vi "test6-AsyncMessageWithReplyWithError.vi"(8 "error in (no error)":errorcluster, 11 "TestCase in":refnum<class "testcase-CSMMessage.lvclass">) -> (0 "error out":errorcluster, 3 "TestCase out":refnum<class "testcase-CSMMessage.lvclass">)   [LabVIEW 2017, in "testcase-CSMMessage.lvclass"]
uses:
  testcase-CSMMessage.lvclass
  948582eb-d69d-4bf1-bb36-25d021f5d5c5.vi
  src/user.lib/_NEVSTOP/Communicable State Machine(CSM)/AdvanceAPI/CSM - Make String Arguments Safe.vi
  src/user.lib/_NEVSTOP/Communicable State Machine(CSM)/AdvanceAPI/CSM - Keywords.vi
  <vilib>/addons/_JKI Toolkits/VI Tester/TestCase.llb/TestCase.lvclass
  src/user.lib/_NEVSTOP/Communicable State Machine(CSM)/Communicable State Machine.lvlib
  C:/Program Files (x86)/National Instruments/LabVIEW 2017/vi.lib/addons/_JKI Toolkits/VI Tester/TestCase.llb/TestCase.lvclass
panel:
  out "Loop Count":i32
  out "concatenated string":string
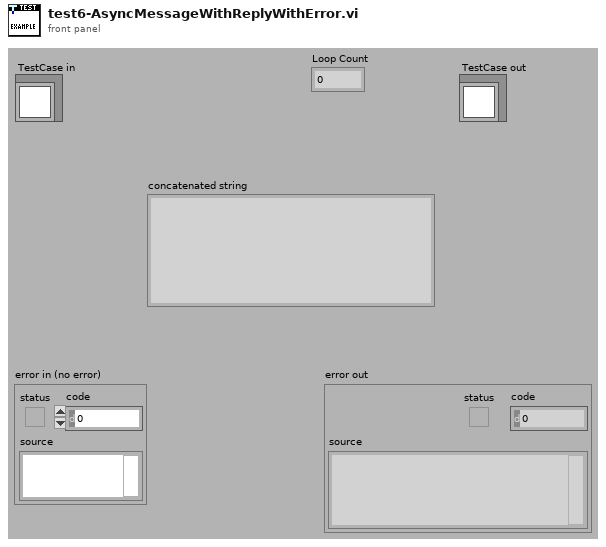
[diagram p1: front panel]
types:
  T1 = cluster{"Arguments":string, "Response":string, "error":errorcluster}
  T2 = cluster{"status":bool, "code":bool, "source":bool}
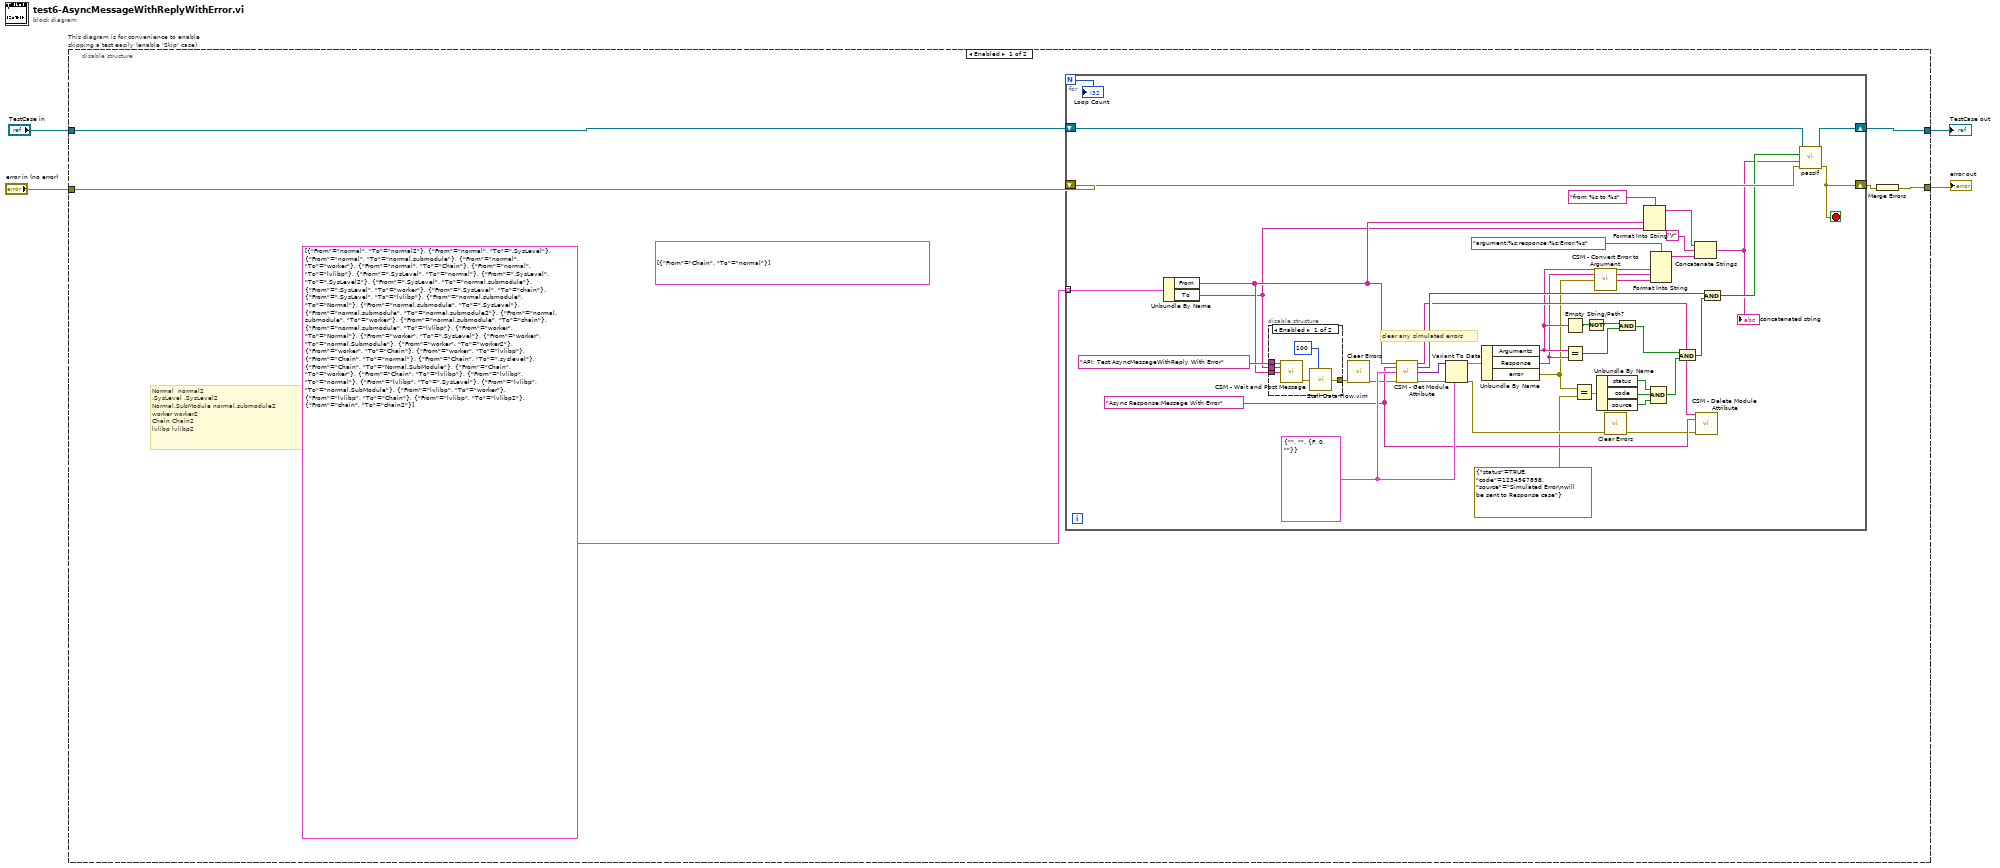
[diagram p0: block diagram]
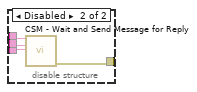
[diagram p2: hidden frame]
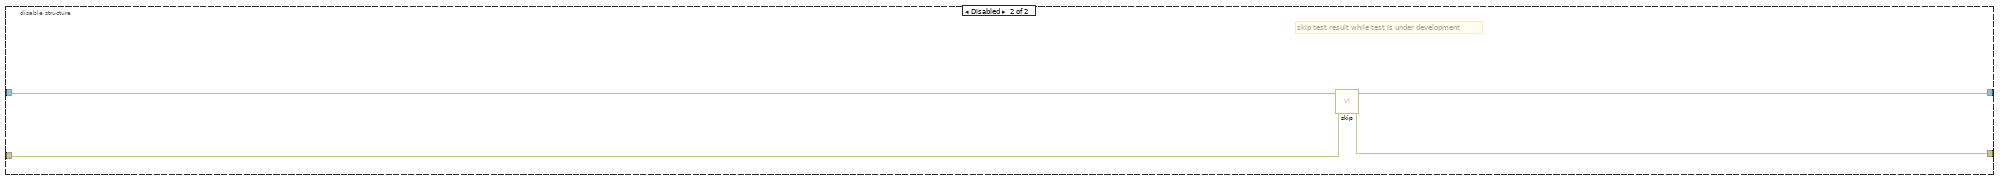
[diagram p3: hidden frame]
diagram:
  n1 = disable-structure "This diagram is for convenience to enable skipping a test easily (enable 'Skip' case)" shown="Enabled" {
    disable-tunnel: "TestCase in" -> [w10 w66]
    disable-tunnel: [w9 w64] -> w1
    disable-tunnel: [w6 w65] -> w3
    disable-tunnel: "error in (no error)" -> [w7 w63]
    frame Enabled {
      (unwired) cluster{"From":string, "To":string}[] [{"From"="Chain", "To"="normal"}]
      # "Normal  normal2\n.SysLevel .SysLevel2\nNormal.SubModule normal.submodule2\nworker worker2\nChain Chain2\nlvlibp lvlibp2"
      n2 = for {
        N -> [w11]
        tunnel: cluster{"From":string, "To":string}[] [{"From"="normal", "To"="normal2"}, {"From"="normal", "To"=".SysLevel"}, {"From"="normal", "To"="normal.submodule"}, {"From"="normal", "To"="worker"}, {"From"="normal", "To"="Chain"}, {"From"="normal", "To"="lvlibp"}, {"From"=".SysLevel", "To"="normal"}, {"From"=".SysLevel", "To"=".SysLevel2"}, {"From"=".SysLevel", "To"="normal.submodule"}, {"From"=".SysLevel", "To"="worker"}, {"From"=".SysLevel", "To"="chain"}, {"From"=".SysLevel", "To"="lvlibp"}, {"From"="normal.submodule", "To"="Normal"}, {"From"="normal.submodule", "To"=".SysLevel"}, {"From"="normal.submodule", "To"="normal.submodule2"}, {"From"="normal.submodule", "To"="worker"}, {"From"="normal.submodule", "To"="chain"}, {"From"="normal.submodule", "To"="lvlibp"}, {"From"="worker", "To"="Normal"}, {"From"="worker", "To"=".SysLevel"}, {"From"="worker", "To"="normal.Submodule"}, {"From"="worker", "To"="worker2"}, {"From"="worker", "To"="Chain"}, {"From"="worker", "To"="lvlibp"}, {"From"="Chain", "To"="normal"}, {"From"="Chain", "To"=".syslevel"}, {"From"="Chain", "To"="Normal.SubModule"}, {"From"="Chain", "To"="worker"}, {"From"="Chain", "To"="lvlibp"}, {"From"="lvlibp", "To"="normal"}, {"From"="lvlibp", "To"=".SysLevel"}, {"From"="lvlibp", "To"="normal.SubModule"}, {"From"="lvlibp", "To"="worker"}, {"From"="lvlibp", "To"="Chain"}, {"From"="lvlibp", "To"="lvlibp2"}, {"From"="chain", "To"="chain2"}] -> [w41] mode=indexing
        shift-right: [w51] -> w9
        shift-left: w10 -> [w52]
        shift-right: [w23] -> w8
        shift-left: w7 -> [w50]
        stop <- w23 stop-if-true
        w47 = T1 {"Arguments"="", "Response"="", "error"={"status"=FALSE, "code"=0, "source"=""}}
        w38 = "Async Response:Message With Error" ("State")
        # "clear any simulated errors"
        n3 = Unbundle By Name(w41) -> ("From"=w15:string, "To"=w14:string)
        n4 = disable-structure shown="Enabled" {
          disable-tunnel: "API: Test AsyncMessageWithReply With Error" ("State") -> [w58 w62]
          disable-tunnel: w15 -> [w57 w60]
          disable-tunnel: w14 -> [w56 w61]
          disable-tunnel: [w53 w59] -> w12
          frame Enabled {
            n5 = call "CSM - Wait and Post Message.vi"("State"=w58, "Arguments (\"\")"=w56, "Target Module"=w57) -> ("error out"=w54:errorcluster)  [unwired: 12 in]
            n6 = call "Stall Data Flow.vim"("value in"=w54, "milliseconds to wait"=u32 100) -> ("value out"=w53:errorcluster)  [unwired: 1 out]
          }
          frame Disabled {
            n7 = call "CSM - Wait and Send Message for Reply.vi"("State"=w62, "Arguments (\"\")"=w61, "Target Module"=w60) -> ("error out"=w59:errorcluster)  [unwired: 10 in, 2 out]
          }
        }
        n8 = call <vilib>:"Clear Errors.vi"("error in (no error)"=w12) -> ("error out"=w13:errorcluster)  [unwired: 5 in, 1 out]
        n9 = call "CSM - Get Module Attribute.vi"("CSM Name"=w15, "Attribute"=w38, "Default Value (Empty Variant)"=w47, "Error In"=w13) -> ("CSM Name (Dup)"=w39:string, "Found"=w44:bool, "Value"=w46:variant, "error out"=w48:errorcluster)  [unwired: 7 in, 1 out]
        n10 = Variant To Data(error in=w48, type=w47, Variant=w46) -> (data=w45:T1, error out=w25:errorcluster)
        n11 = Unbundle By Name(w45) -> ("Arguments"=w33:string, "Response"=w32:string, "error"=w22:errorcluster)
        n12 = Empty String/Path?(string/path=w33) -> (empty?=w37:bool)
        n13 = Equal?(x=w33, y=w32) -> (x = y?=w35:bool)
        n14 = Equal?(x=w22, y=errorcluster {"status"=TRUE, "code"=1234567898, "source"="Simulated Error\nwill be sent to Response case"} ("error out")) -> (x = y?=w20:T2)
        n15 = Not(x=w37) -> (.not. x?=w36:bool)
        n16 = call "CSM - Convert Error to Argument.vi"("Error"=w22) -> ("Argument"=w31:string)  [unwired: 4 in]
        n17 = Unbundle By Name(w20) -> ("status"=w19:bool, "code"=w18:bool, "source"=w17:bool)
        n18 = call <vilib>:"Clear Errors.vi"("error in (no error)"=w25) -> ("error out"=w24:errorcluster)  [unwired: 5 in, 1 out]
        n19 = And(x=w36, y=w35) -> (x .and. y?=w34:bool)
        n20 = Format Into String(format string="from %s to %s", w15, w14) -> (resulting string=w27:string)  [unwired: 2 in, 1 out]
        n21 = Format Into String(format string="argument:%s;response:%s;Error:%s", w33, w32, w31) -> (resulting string=w30:string)  [unwired: 2 in, 1 out]
        n22 = Compound Arithmetic op=AND(w19, w18, w17) -> (w16:bool)
        n23 = And(x=w34, y=w16) -> (x .and. y?=w43:bool)
        n24 = Concatenate Strings(w27, "\r", w30) -> (w28:string)
        "concatenated string" <- w28
        n25 = call "CSM - Delete Module Attribute.vi"("CSM Name"=w39, "Attribute"=w38, "Error In"=w24) -> ()  [unwired: 9 in, 4 out]
        n26 = And(x=w44, y=w43) -> (x .and. y?=w42:bool)
        n27 = call-dynamic "passIf.vi"("error in (no error)"=w50, "message (\"\")"=w28, "pass"=w42, "TestCase in"=w52) -> ("error out"=w23:errorcluster, "TestCase out"=w51:refnum<class "testcase-CSMMessage.lvclass">)  [unwired: 6 in]
        "Loop Count" <- w11
      }
      n28 = Merge Errors(w8) -> (w6:errorcluster)
    }
    frame Disabled {
      # "skip test result while test is under development"
      n29 = call <vilib>:"skip.vi"("error in (no error)"=w63, "TestCase in"=w66) -> ("error out"=w65:errorcluster, "TestCase out"=w64:refnum<class "testcase-CSMMessage.lvclass">)  [unwired: 8 in]
    }
  }
  "error out" <- w3
  "TestCase out" <- w1
